vi "Start-acquisition-hardware.vi"(8 "error in":errorcluster, 11 "Config. params in":refnum<data-value>) -> (0 "error IO":errorcluster, 3 "Config. params":refnum<data-value>)   [LabVIEW 2013, in "CameraVision.lvlib" / "CV-Configuration.lvclass"]
uses:
  CV-Configuration.lvclass
  UI/Module-states.ctl
  CV-Configuration.lvclass/CV-Configuration.ctl
  Read Framegrabber DLL file.vi
  Read BoardHandle.vi
  Read Camport array.vi
  Read DMA adresses.vi
  Write Camera status.vi
  Write Grabber status.vi
  UI/CV-UI.lvclass
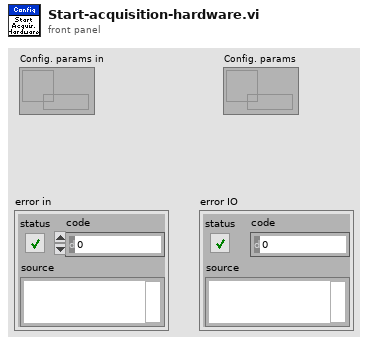
[diagram p1: front panel]
types:
  T1 = typedef "CameraVision.lvlib/CV-UI.lvclass/Module-states.ctl" = enum16{"Inactive", "Active", "Data-loss", "Error", "Simulation", "Synchronizing", "Initialized", "Released"}
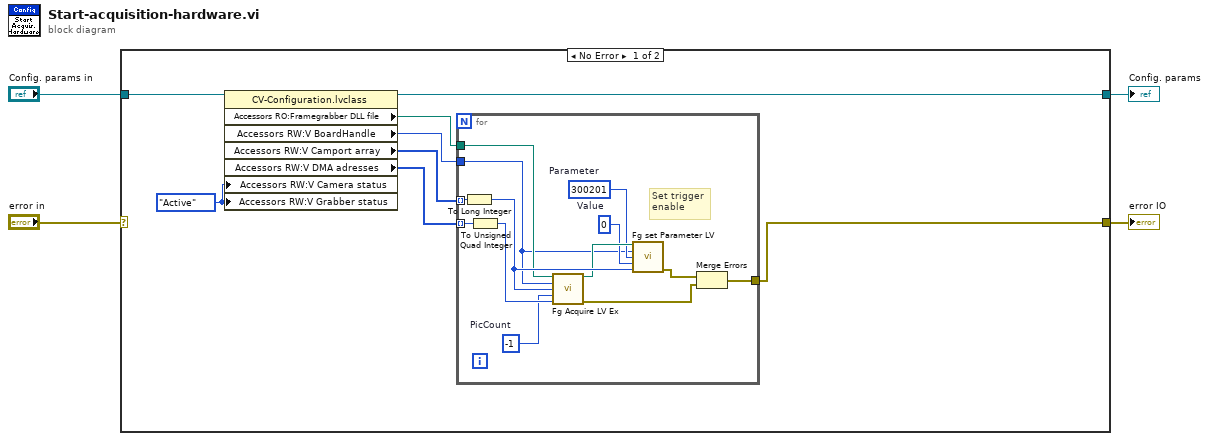
[diagram p0: block diagram]
diagram:
  n1 = case shown="No Error" "error in" {
    selector: "error in" -> [_ w27]
    tunnel: [w5 w27] -> w4
    tunnel: "Config. params in" -> [w12 w26]
    tunnel: [w11 w26] -> w1
    frame No Error {
      w9 = Module-states."Active" ("Camera status")
      n2 = property class="CV-Configuration.lvclass"(reference=w12, "Accessors RW:V Camera status"=w9, "Accessors RW:V Grabber status"=w9) -> (reference out=w11:refnum<data-value>, "Accessors RO:Framegrabber DLL file"=w8:path, "Accessors RW:V BoardHandle"=w10:u64, "Accessors RW:V Camport array"=w7:u32[], "Accessors RW:V DMA adresses"=w6:i64[])  [unwired: 1 in, 1 out]
      n3 = for {
        tunnel: w8 -> [w14]
        tunnel: w10 -> [w13]
        tunnel: w7 -> [w25] mode=indexing
        tunnel: w6 -> [w24] mode=indexing
        tunnel: [w17] -> w5
        w15 = u32 0  # Value
        w16 = 300201  # Parameter
        w22 = -1  # PicCount
        # "Set trigger \nenable"
        n4 = To Long Integer(number=w25) -> (32bit integer=w21:i32)
        n5 = To Unsigned Quad Integer(1:w24) -> (0:w23:u64)
        n6 = call <userlib>:"Fg Acquire LV Ex.vi"("dll path in"=w14, "FgAddr"=w13, "CamPort"=w21, "PicCount"=w22, "DmaAddr"=w23) -> ("dll path out"=w20:path, "error out"=w18:errorcluster)  [unwired: 8 in, 1 out]
        n7 = call <userlib>:"Fg set Parameter LV.vi"("dll path in"=w20, "FgAddr"=w13, "Parameter"=w16, "Value"=w15, "CamPort"=w21) -> ("error out"=w19:errorcluster)  [unwired: 8 in, 2 out]
        n8 = Merge Errors(w19, w18) -> (w17:errorcluster)
      }
    }
    frame Error {
    }
  }
  "error IO" <- w4
  "Config. params" <- w1
